vi "Write TDMS.vi"(4 "Append Index":i32, 6 "Commands":string, 8 "error in (no error)":errorcluster, 9 "Notes":string, 10 "Data (Dictionary)":T1[](array[typedef]), 11 "path":path) -> (0 "error out":errorcluster, 3 "path out":path)   [LabVIEW 2016, in "Data.TDMS.lvclass"]
uses:
  Data.TDMS.lvclass
  Data/Data.lvclass
  Data/Typedefs/Dictionary--cluster.ctl
panel:
  in  "Append? [F] 2":bool
  # "Not used:"
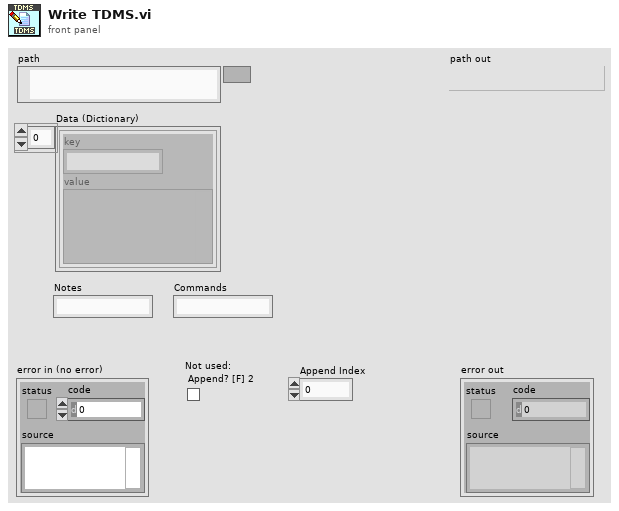
[diagram p1: front panel]
types:
  T1 = typedef "Data.lvclass/Dictionary--cluster.ctl" = cluster{"key":string, "value":variant}
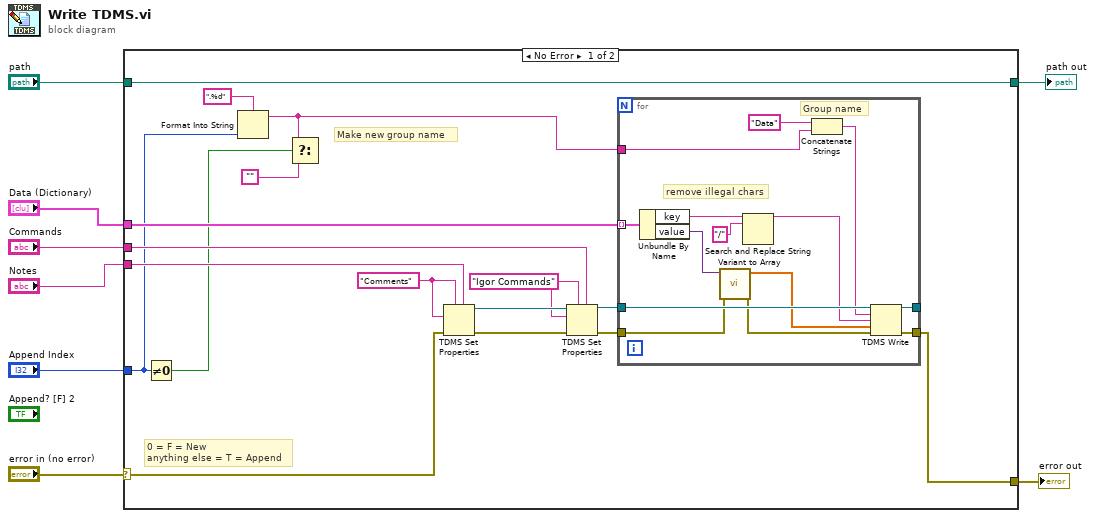
[diagram p0: block diagram]
diagram:
  n1 = case shown="No Error" "error in (no error)" {
    selector: "error in (no error)" -> [w15 w41]
    tunnel: [w21 w41] -> w4
    tunnel: "Append Index" -> [w13 _]
    tunnel: "path" -> [w11 w40]
    tunnel: "Notes" -> [w16 _]
    tunnel: "Commands" -> [w17 _]
    tunnel: "Data (Dictionary)" -> [w18 _]
    tunnel: [w11 w40] -> w5
    frame No Error {
      w20 = "Igor Commands" ("attrib name")
      w19 = "Comments" ("attrib name")
      # "Make new group name"
      # "0 = F = New\nanything else = T = Append"
      n2 = Not Equal To 0?(x=w13) -> (x != 0?=w14:bool)
      n3 = Format Into String(format string=".%d", w13) -> (resulting string=w9:string)  [unwired: 2 in, 1 out]
      n4 = Select(t=w9, s=w14, f="") -> ()  [unwired: 1 out]
      n5 = TDMS Set Properties(5:w16, 7:w19, 8:w15, 10:w19) -> (0:w24:errorcluster, 3:w25:refnum<k34>)  [unwired: 2 in, 2 out]
      n6 = TDMS Set Properties(5:w17, 7:w20, 8:w24, 10:w20, 11:w25) -> (0:w23:errorcluster, 3:w22:refnum<k34>)  [unwired: 1 in, 2 out]
      n7 = for {
        tunnel: w18 -> [w34] mode=indexing
        tunnel: w23 -> [w31]
        tunnel: w22 -> [w38]
        tunnel: [w37] -> w21
        tunnel: [w36] -> _
        tunnel: w9 -> [w27]
        # "Group name"
        # "remove illegal chars"
        n8 = Unbundle By Name(w34) -> ("key"=w35:string, "value"=w30:variant)
        n9 = call "Variant to Array.vi"("error in (no error)"=w31, "Data (Variant)"=w30) -> ("error out"=w32:errorcluster, "1D Array"=w29:dbl[])  [unwired: 7 in, 1 out]
        n10 = Search and Replace String(input string=w35, search string="/") -> (result string=w33:string)  [unwired: 6 in, 3 out]
        n11 = Concatenate Strings("Data" ("group name in (Untitled)"), w27) -> (w26:string)
        n12 = TDMS Write(0:w38, 5:w26, 7:w33, 9:w29, 11:w32) -> (4:w36:refnum<k34>, 15:w37:errorcluster)  [unwired: 1 in, 2 out]
      }
    }
    frame Error {
    }
  }
  "error out" <- w4
  "path out" <- w5
